vi "Create Timing (cluster).vi"(7 "id (0)":i32, 8 "error in (no error)":errorcluster, 10 "cycle timing":T1, 11 "Timing in":refnum<class "Timing.lvclass">) -> (0 "error out":errorcluster, 3 "Timing":refnum<class "Timing.lvclass">)   [LabVIEW 2019, in "DSF Core.lvlib" / "Timing.lvclass"]
uses:
  Timing.lvclass
  Typedefs/DSF Timing Info.ctl
  DSF Core.lvlib
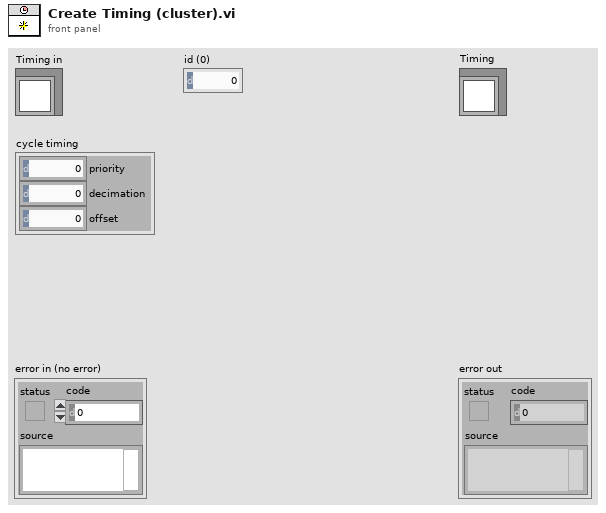
[diagram p1: front panel]
types:
  T1 = typedef "DSF Core.lvlib/DSF Timing Info.ctl" = cluster{"priority":u64, "decimation":u64, "offset":u64}
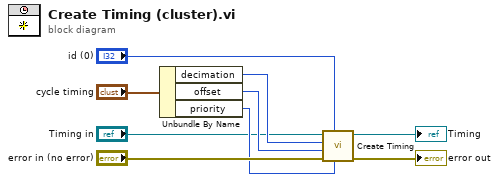
[diagram p0: block diagram]
diagram:
  n1 = Unbundle By Name("cycle timing") -> ("decimation"=w4:u64, "offset"=w5:u64, "priority"=w2:u64)
  n2 = call "Create Timing.vi"("priority"=w2, "id (0)"="id (0)", "error in (no error)"="error in (no error)", "offset"=w5, "decimation"=w4, "Timing in"="Timing in") -> ("error out"=→"error out":errorcluster, "Timing out"=→"Timing":refnum<class "Timing.lvclass">)  [unwired: 4 in]
